vi "Write Keys.vi"(8 "error in (no error)":errorcluster) -> (0 "error out":errorcluster, 3 "text":string)   [LabVIEW 2017, in "labview-config-library.lvclass"]
uses:
  labview-config-library.lvclass
  INI-Static-Variable-Support/LabVIEW-Config/LabVIEW-Config.lvclass
  INI-Static-Variable-Support/LabVIEW-Config/Write Key (Boolean).vi
  INI-Static-Variable-Support/LabVIEW-Config/Write Key (I32).vi
  INI-Static-Variable-Support/LabVIEW-Config/Write Key (U32).vi
  INI-Static-Variable-Support/LabVIEW-Config/Write Key (DBL).vi
  INI-Static-Variable-Support/LabVIEW-Config/Write Key (String).vi
panel:
  in  "Config":T1={"String"="Goodbye moon", "Boolean"=FALSE, "Int"=-514, "Uint"=92834, "Float"=0.0012, "Raw"="Foo bar"}
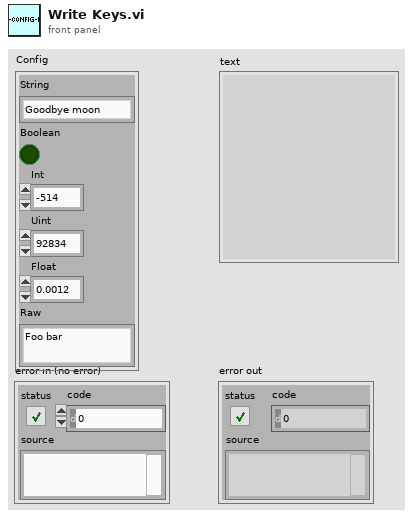
[diagram p1: front panel]
types:
  T1 = cluster{"String":string, "Boolean":bool, "Int":i32, "Uint":u32, "Float":dbl, "Raw":string}
  T2 = typedef "LabVIEW-Config.lvlib/LabVIEW-Config.lvclass/Config.ctl" = cluster{"Path":path, "Lines":string[], "Tokens":T3[], "Modified?":bool, "Cache":cluster{"Valid?":bool, "Key Information":T4[]}}
  T3 = typedef "LabVIEW-Config.lvlib/LabVIEW-Config.lvclass/LineToken.ctl" = enum8{"comment", "section", "key", "more"}
  T4 = typedef "LabVIEW-Config.lvlib/LabVIEW-Config.lvclass/KeyInfo.ctl" = cluster{"Key Indexes":cluster{"Indexes":i32[]}[], "Session Found?":bool, "Key found?":bool, "Session Index":i32}
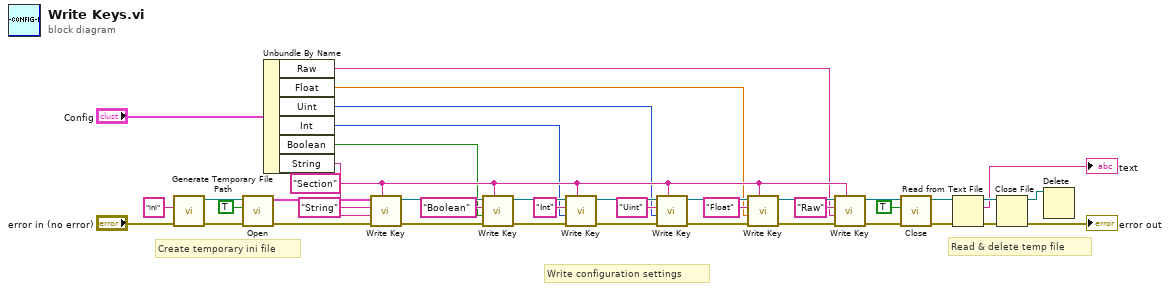
[diagram p0: block diagram]
diagram:
  w18 = "Section" ("Section Name")
  # "Read & delete temp file"
  # "Write configuration settings"
  # "Create temporary ini file"
  n1 = call <vilib>:"Generate Temporary File Path.vi"("error in (no error)"="error in (no error)", "Temporary File Extension (tmp)"="ini") -> ("error out"=w15:errorcluster, "Unique Temporary File Path"=w14:path)  [unwired: 8 in]
  n2 = call "Open.vi"("error in (no error)"=w15, "Create if not exists? (T)"=TRUE, "Path"=w14) -> ("error out"=w38:errorcluster, "Config"=w39:T2)  [unwired: 5 in, 2 out]
  n3 = Unbundle By Name("Config") -> ("Raw"=w7:string, "Float"=w8:dbl, "Uint"=w9:u32, "Int"=w10:i32, "Boolean"=w11:bool, "String"=w12:string)
  n4 = call-poly "Write Key.vi"("Section Name"=w18, "error in (no error)"=w38, "Value"=w12, "Key Name"="String", "Config in"=w39) -> ("error out"=w35:errorcluster, "Config out"=w34:refnum<class "LabVIEW-Config.lvclass">)  [unwired: 4 in, 1 out]
  n5 = call-poly "Write Key.vi"("Section Name"=w18, "error in (no error)"=w35, "Value"=w11, "Key Name"="Boolean", "Config in"=w34) -> ("error out"=w33:errorcluster, "Config out"=w31:refnum<class "LabVIEW-Config.lvclass">)  [unwired: 4 in, 1 out]
  n6 = call-poly "Write Key.vi"("Section Name"=w18, "error in (no error)"=w33, "Value"=w10, "Key Name"="Int", "Config in"=w31) -> ("error out"=w32:errorcluster, "Config out"=w26:refnum<class "LabVIEW-Config.lvclass">)  [unwired: 4 in, 1 out]
  n7 = call-poly "Write Key.vi"("Section Name"=w18, "error in (no error)"=w32, "Value"=w9, "Key Name"="Uint", "Config in"=w26) -> ("error out"=w27:errorcluster, "Config out"=w23:refnum<class "LabVIEW-Config.lvclass">)  [unwired: 4 in, 1 out]
  n8 = call-poly "Write Key.vi"("Section Name"=w18, "error in (no error)"=w27, "Value"=w8, "Key Name"="Float", "Config in"=w23) -> ("error out"=w24:errorcluster, "Config out"=w20:refnum<class "LabVIEW-Config.lvclass">)  [unwired: 4 in, 1 out]
  n9 = call-poly "Write Key.vi"("Section Name"=w18, "error in (no error)"=w24, "Value"=w7, "Key Name"="Raw", "Config in"=w20) -> ("error out"=w21:errorcluster, "Config out"=w19:refnum<class "LabVIEW-Config.lvclass">)  [unwired: 4 in, 1 out]
  n10 = call "Close.vi"("error in (no error)"=w21, "Write if modified? (T)"=TRUE, "Config"=w19) -> ("error out"=w16:errorcluster, "Path"=w5:path)  [unwired: 7 in]
  n11 = Read from Text File(file (use dialog)=w5, error in=w16) -> (refnum out=w3:refnum<file>, text=→"text":string, error out=w6:errorcluster)  [unwired: 2 in, 1 out]
  n12 = Close File(refnum=w3, error in=w6) -> (path=w2:path, error out=→"error out":errorcluster)
  n13 = Delete(path (use dialog)=w2) -> ()  [unwired: 4 in, 3 out]
